vi "SiosIfmUSBDeviceSerial.vi"(1 "order number in the list of devices, that was created by the function IfmSearchUSBDevices":i32) -> (0 "Serial Number of Device":i32)   [LabVIEW 2009]
uses:
  siosifm.dll
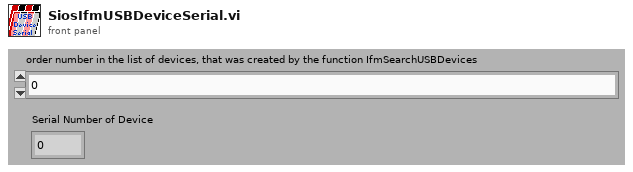
[diagram p1: front panel]
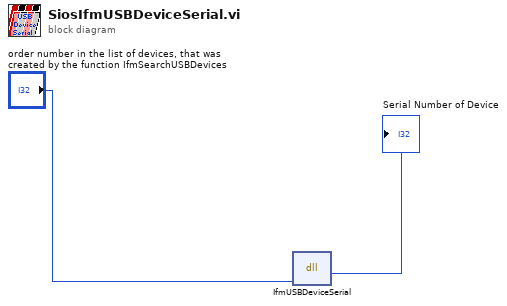
[diagram p0: block diagram]
diagram:
  n1 = dll-call lib="C:/WORK/Artem/RE-10/SIOS_IfmDLL/siosifm.dll" fn="IfmUSBDeviceSerial"("uniqueld"="order number in the list of devices, that was created by the function IfmSearchUSBDevices") -> ("serial number"=→"Serial Number of Device":i32)  [unwired: 4 in, 2 out]
